vi "Start.vi"(6 "ms timeout (if waiting)":i32=-1, 8 "error in (no error)":errorcluster, 9 "Wait Until Shutdown? (F)":bool, 11 "SMO":refnum<class "SMO.lvclass">) -> (0 "error out":errorcluster, 3 "SMO out":refnum<class "SMO.lvclass">)   [LabVIEW 2021, in "smo.lvlib" / "SMO.lvclass"]
doc: "In the default mode (when <b>Wait Until Shutdown?</b> is False), this method will start (launch asynchronously) the registered processes.\n\nIf <b>Wait Until Shutdown?</b> is True, then this method is blocking (process launch is synchronous) until either the stop method is invoked or <b>ms timeout</b> is reached.\n\nNote 01: This method is overridable by descendant\nNote 02: When overridden, Call Parent Method is required\n\n---------------------------------------------------------------\nJKI State Machine Objects™\nhttp://jki.net/state-machine-objects/\nCopyright (C) 2005-2015, JKI <info@jki.net>\nALL RIGHTS RESERVED"
uses:
  SMO.lvclass
  Typedefs/SMOState --Enum.ctl
  SMO.lvclass/SMO.ctl
panel:
  # "For instructions on how to use the JKI State Machine Objects, examples and video tutorials, visit:\nhttp://jki.net/state-machine-objects/\n\nJKI State Machine Objects™\nhttp://jki.net/state-machine-objects/\nCopyright (C) 2005-2015, JKI <info@jki.net>\nALL RIGHTS RESERVED"
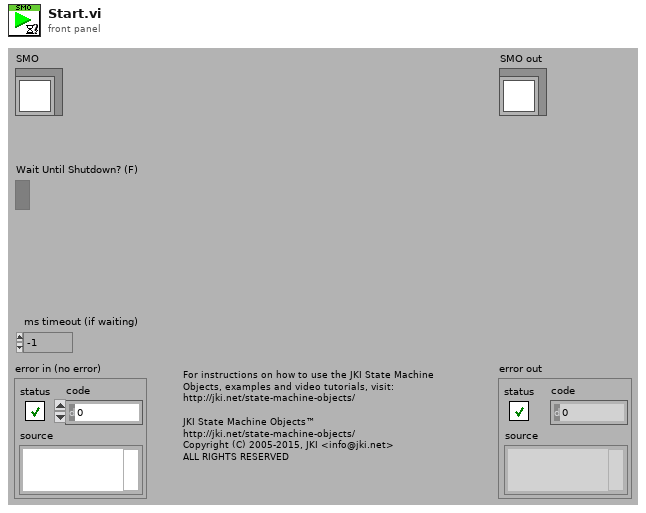
[diagram p1: front panel]
types:
  T1 = typedef "smo.lvlib/SMO.lvclass/SMOState --Enum.ctl" = enum16{"unknown", "Created", "Started", "Stopped"}
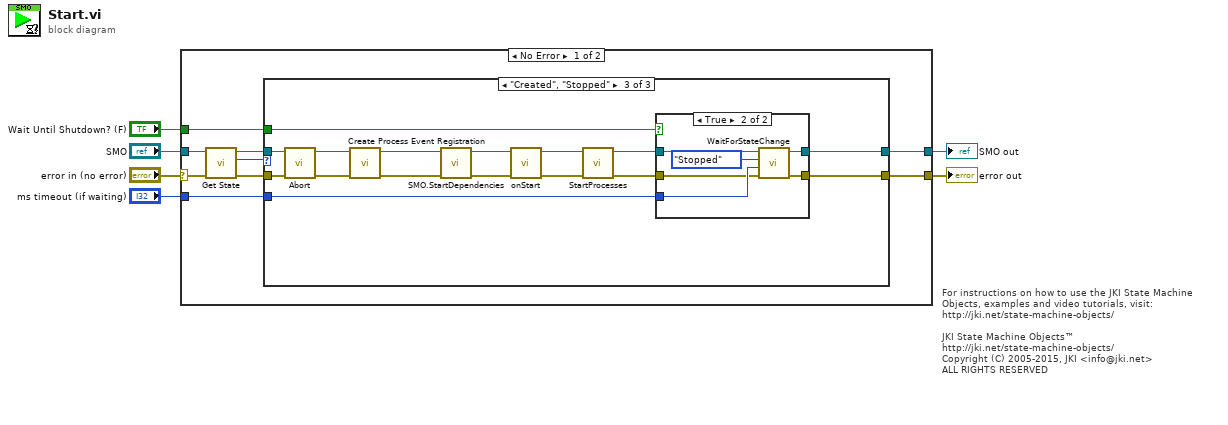
[diagram p0: block diagram]
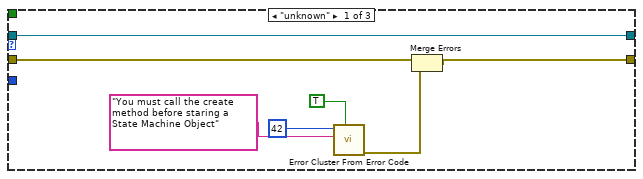
[diagram p2: hidden frame]
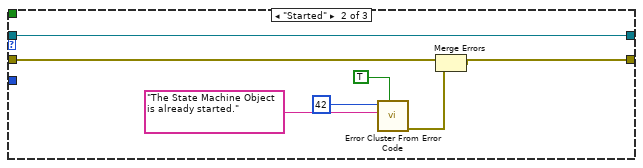
[diagram p3: hidden frame]
diagram:
  # "For instructions on how to use the JKI State Machine Objects, examples and video tutorials, visit:\nhttp://jki.net/state-machine-objects/\n\nJKI State Machine Objects™\nhttp://jki.net/state-machine-objects/\nCopyright (C) 2005-2015, JKI <info@jki.net>\nALL RIGHTS RESERVED"
  n1 = case shown="No Error" "error in (no error)" {
    selector: "error in (no error)" -> [w11 w55]
    tunnel: [w7 w55] -> w5
    tunnel: [w8 w54] -> w3
    tunnel: "SMO" -> [w13 w54]
    tunnel: "Wait Until Shutdown? (F)" -> [w15 _]
    tunnel: "ms timeout (if waiting)" -> [w14 _]
    frame No Error {
      n2 = call "Get State.vi"("error in (no error)"=w11, "SMO"=w13) -> ("error out"=w10:errorcluster, "SMO State"=w9:T1, "SMO out"=w12:refnum<class "SMO.lvclass">)  [unwired: 7 in]
      n3 = case shown="\"Created\", \"Stopped\"" w9 {
        tunnel: [w22 w29 w45] -> w8
        tunnel: [w17 w24 w44] -> w7
        tunnel: w15 -> [_ _ w43]
        tunnel: w14 -> [_ _ w35]
        tunnel: w12 -> [w22 w29 w39]
        tunnel: w10 -> [w18 w25 w38]
        frame "unknown" {
          n4 = call <vilib>:"Error Cluster From Error Code.vi"("show call chain? (False)"=TRUE, "error message (\"\")"="You must call the create method before staring a State Machine Object" ("error message (\"\")"), "error code (0)"=42) -> ("error out"=w16:errorcluster)  [unwired: 6 in]
          n5 = Merge Errors(w18, w16) -> (w17:errorcluster)
        }
        frame "Started" {
          n6 = call <vilib>:"Error Cluster From Error Code.vi"("show call chain? (False)"=TRUE, "error message (\"\")"="The State Machine Object is already started." ("error message (\"\")"), "error code (0)"=42) -> ("error out"=w23:errorcluster)  [unwired: 6 in]
          n7 = Merge Errors(w25, w23) -> (w24:errorcluster)
        }
        frame "Created", "Stopped" {
          n8 = call "Abort.vi"("error in (no error)"=w38, "SMO"=w39) -> ("error out"=w36:errorcluster, "SMO out"=w37:refnum<class "SMO.lvclass">)  [unwired: 8 in]
          n9 = call "Create Process Event Registration.vi"("error in (no error)"=w36, "SMO in"=w37) -> ("error out"=w34:errorcluster, "SMO out"=w32:refnum<class "SMO.lvclass">)  [unwired: 8 in]
          n10 = call "SMO.StartDependencies.vi"("error in (no error)"=w34, "SMO in"=w32) -> ("error out"=w33:errorcluster, "SMO out"=w31:refnum<class "SMO.lvclass">)  [unwired: 8 in]
          n11 = call-dynamic "onStart.vi"("error in (no error)"=w33, "SMO"=w31) -> ("error out"=w30:errorcluster, "SMO out"=w40:refnum<class "SMO.lvclass">)  [unwired: 8 in]
          n12 = call "StartProcesses.vi"("error in (no error)"=w30, "SMO"=w40) -> ("error out"=w41:errorcluster, "SMO out"=w42:refnum<class "SMO.lvclass">)  [unwired: 8 in]
          n13 = case shown="True" w43 {
            tunnel: w42 -> [w47 w51]
            tunnel: [w47 w50] -> w45
            tunnel: w41 -> [w46 w49]
            tunnel: [w46 w52] -> w44
            tunnel: w35 -> [_ w53]
            frame False {
            }
            frame True {
              n14 = call "WaitForStateChange.vi"("error in (no error)"=w49, "timeout in ms (-1)"=w53, "State (unknown: Any state change)"=SMOState_--Enum."Stopped", "SMO in"=w51) -> ("error out"=w52:errorcluster, "SMO out"=w50:refnum<class "SMO.lvclass">)  [unwired: 5 in, 1 out]
            }
          }
        }
      }
    }
    frame Error {
    }
  }
  "error out" <- w5
  "SMO out" <- w3
